vi "Modbus Master.vi"(0 "starting address":u16 caption="起始地址", 1 "error in":errorcluster, 5 "holding register values":u16[](array[numeric]) caption="写入保持寄存器的值", 9 "读取写入选择":string(combo), 11 "Unit ID":u8=1) -> (3 "error out":errorcluster, 4 "仪器状态":u16[](array[numeric]), 6 "试剂余量":u16[](array[numeric]), 8 "输出":T1, 10 "各参数测量间隔":u16[](array[numeric]), 14 "校准点信息":u16[](array[numeric]), 15 "关键参数":u16[](array[numeric]))   [LabVIEW 2016, in "数据传输系统.lvlib"]
uses:
  <vilib>/NI/Modbus Library/API/Modbus API.lvclass/Modbus API.ctl
  <vilib>/NI/Modbus Library/Transmission Data Unit/Transmission Data Unit.lvclass/Transmission Data Unit.ctl
  <vilib>/NI/Modbus Library/API/Master/Set Unit ID.vi
  <vilib>/NI/Modbus Library/Transmission Data Unit/Write Unit ID.vi
  <vilib>/NI/Modbus Library/API/Read Transmission Data Unit.vi
  <vilib>/NI/Modbus Library/API/Write Transmission Data Unit.vi
  <vilib>/NI/Modbus Library/API/master/Modbus Master.lvclass
  E:/Program Files (x86)/National Instruments/LabVIEW 2016/vi.lib/NI/Modbus Library/API/Modbus API.lvclass
  <vilib>/NI/Modbus Library/API/Wrapper/Create TCP Master.vi
  <vilib>/NI/Modbus Library/API/Modbus API.lvclass
  <vilib>/NI/Modbus Library/API/Wrapper/API Main.lvlib
panel:
  out "系统信息":u16[](array[numeric]) caption="校准点信息"
  out "告警信息":u16[](array[numeric]) caption="校准点信息"
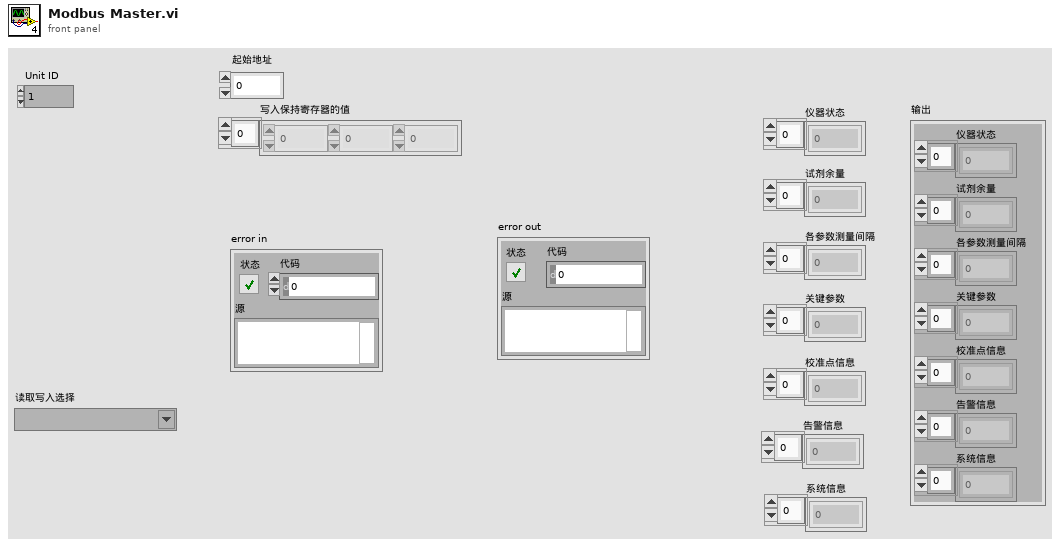
[diagram p1: front panel]
types:
  T1 = cluster{"仪器状态":u16[], "试剂余量":u16[], "各参数测量间隔":u16[], "关键参数":u16[], "校准点信息":u16[], "告警信息":u16[], "系统信息":u16[]}
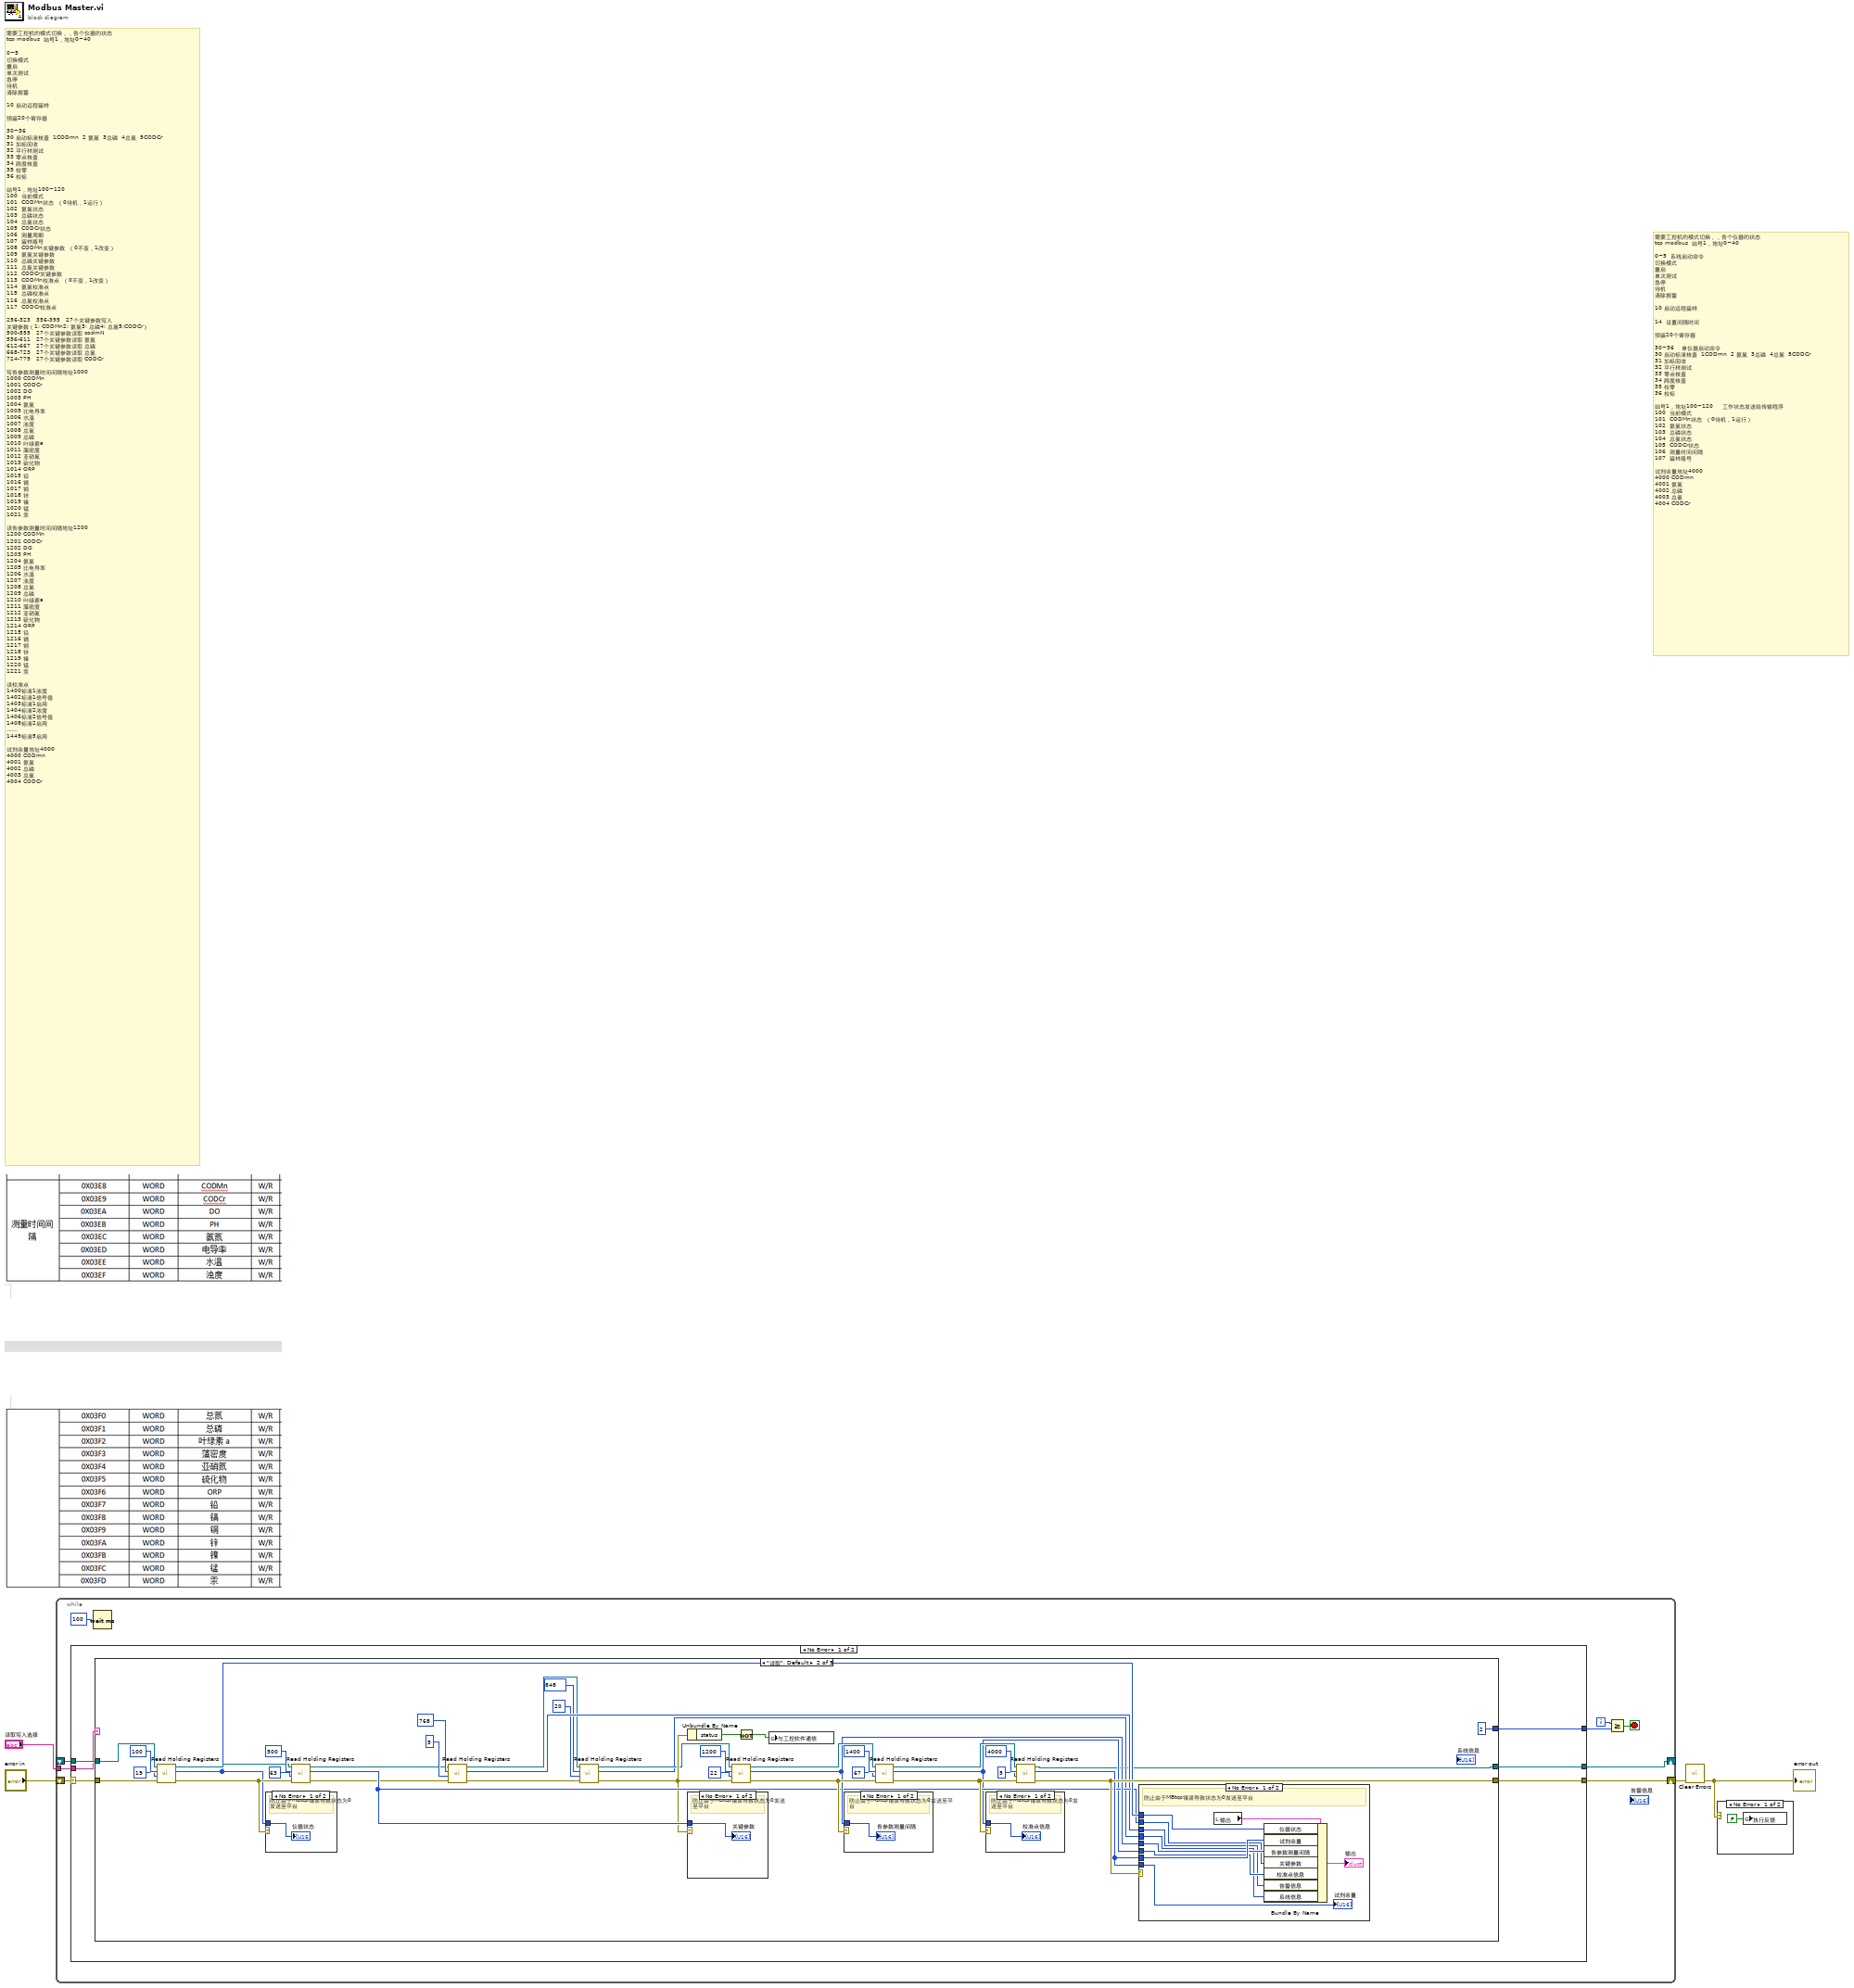
[diagram p0: block diagram]
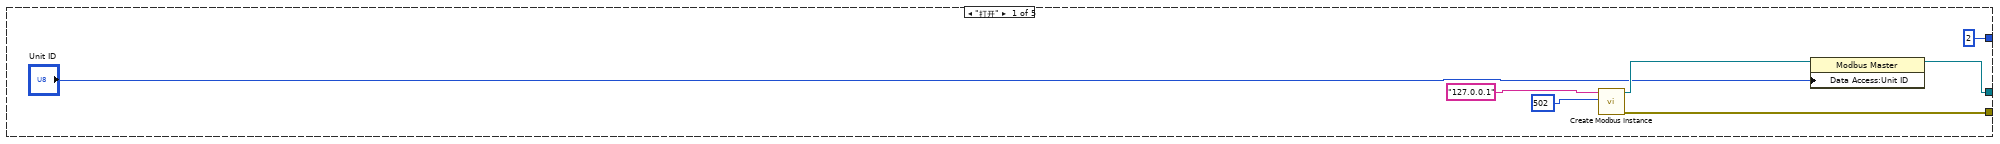
[diagram p3: hidden frame]
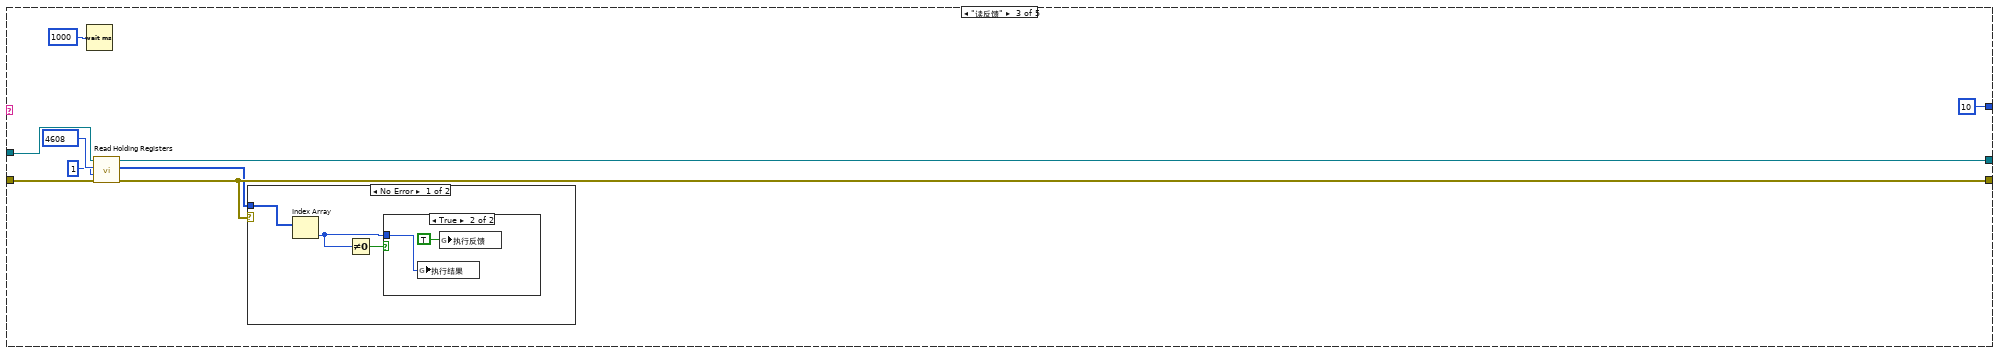
[diagram p9: hidden frame]
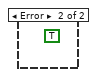
[diagram p11: hidden frame]
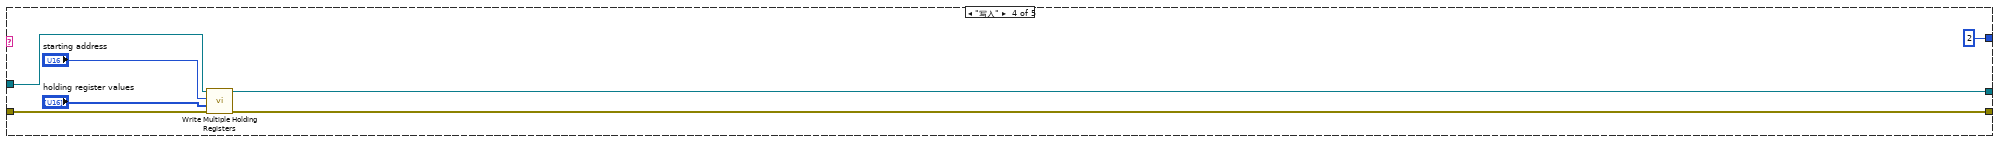
[diagram p12: hidden frame]
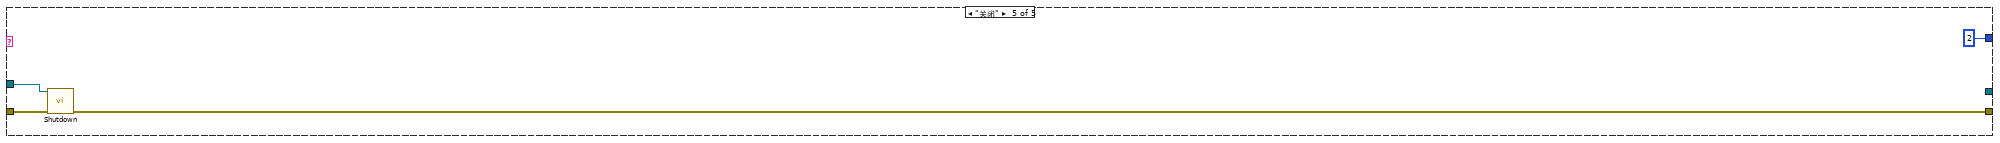
[diagram p13: hidden frame]
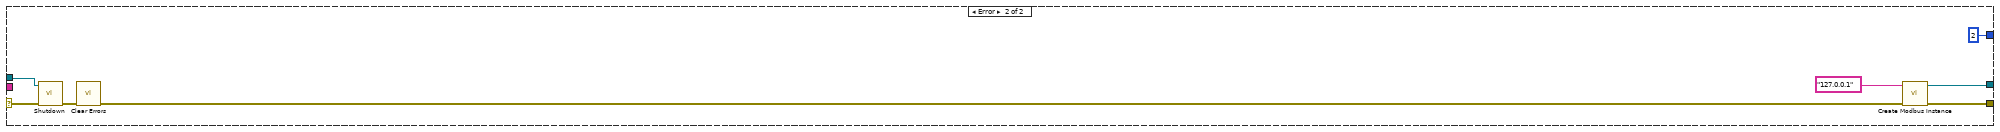
[diagram p14: hidden frame]
diagram:
  # "需要工控机的模式切换，，各个仪器的状态\ntcp modbus  站号1，地址0~40\n\n0~5  系统启动命令\n切换模式\n重启\n单次测试\n急停\n待机\n清除报警\n\n10 启动远程留样\n\n14  设置间隔时间\n\n预留20个寄存器\n\n30~36    单仪器启动命令\n30 启动标液核查  1CODmn  2 氨氮  3总磷  4总氮  5CODCr\n31 加标回收\n32 平行样测试\n33 零点核查\n34 跨度核查\n35 校零\n36 校标\n\n站号1，地址100~120     工作状态发送给传输程序\n100  当前模式\n101  CODMn状态  （0待机，1运行）\n102  氨氮状态\n103  总磷状态\n104  总氮状态\n105  CODCr状态\n106  测量时间间隔\n107  留样瓶号\n\n试剂余量地址4000\n4000 CODmn\n4001 氨氮\n4002 总磷\n4003 总氮\n4004 CODCr"
  # "需要工控机的模式切换，，各个仪器的状态\ntcp modbus  站号1，地址0~40\n\n0~5\n切换模式\n重启\n单次测试\n急停\n待机\n清除报警\n\n10 启动远程留样\n\n预留20个寄存器\n\n30~36\n30 启动标液核查  1CODmn  2 氨氮  3总磷  4总氮  5CODCr\n31 加标回收\n32 平行样测试\n33 零点核查\n34 跨度核查\n35 校零\n36 校标\n\n站号1，地址100~120\n100  当前模式\n101  CODMn状态  （0待机，1运行）\n102  氨氮状态\n103  总磷状态\n104  总氮状态\n105  CODCr状态\n106  测量周期\n107  留样瓶号\n108  CODMn关键参数  （0不变，1改变）\n109  氨氮关键参数\n110  总磷关键参数\n111  总氮关键参数\n112  CODCr关键参数\n113  CODMn校准点  （0不变，1改变）\n114  氨氮校准点\n115  总磷校准点\n116  总氮校准点\n117  CODCr校准点\n\n256-323   356-395   27个关键参数写入\n关键参数（1: CODMn2: 氨氮3: 总磷4: 总氮5:CODCr） \n500-555   27个关键参数读取 codmN\n556-611   27个关键参数读取 氨氮\n612-667   27个关键参数读取 总磷\n668-723   27个关键参数读取 总氮\n724-779   27个关键参数读取 CODCr\n\n写各参数测量时间间隔地址1000\n1000 CODMn\n1001 CODCr\n1002 DO\n1003 PH\n1004 氨氮\n1005 比电导率\n1006 水温\n1007 浊度\n1008 总氮\n1009 总磷\n1010 叶绿素a\n1011 藻密度\n1012 亚硝氮\n1013 硫化物\n1014 ORP\n1015 铅\n1016 镉\n1017 铜\n1018 锌\n1019 镍\n1020 锰\n1021 汞\n\n读各参数测量时间间隔地址1200\n1200 CODMn\n1201 CODCr\n1202 DO\n1203 PH\n1204 氨氮\n1205 比电导率\n1206 水温\n1207 浊度\n1208 总氮\n1209 总磷\n1210 叶绿素a\n1211 藻密度\n1212 亚硝氮\n1213 硫化物\n1214 ORP\n1215 铅\n1216 镉\n1217 铜\n1218 锌\n1219 镍\n1220 锰\n1221 汞\n\n读校准点\n1400标液1浓度\n1402标液1信号值\n1403标液1启用\n1404标液2浓度\n1406标液2信号值\n1408标液2启用\n......\n1449标液5启用\n\n试剂余量地址4000\n4000 CODmn\n4001 氨氮\n4002 总磷\n4003 总氮\n4004 CODCr"
  n1 = while {
    shift-right: [w7] -> w2
    shift-left: "error in" -> [w11]
    shift-right: [w12] -> _
    shift-left: _ -> [w13]
    tunnel: "读取写入选择" -> [w8]
    i -> [w9]
    stop <- w6 stop-if-true
    n2 = case shown="No Error" w11 {
      selector: w11 -> [w16 w107]
      tunnel: w13 -> [w19 w109]
      tunnel: [w18 w111] -> w12
      tunnel: [w17 w110] -> w7
      tunnel: w8 -> [w15 _]
      tunnel: [w14 2 ("y")] -> w5
      frame No Error {
        n3 = case shown="\"读取\", Default" w15 {
          tunnel: w19 -> [_ w66 w87 w101 w105]
          tunnel: [w23 w27 w85 w100 _] -> w18
          tunnel: [w22 w57 w84 w99 w103] -> w17
          tunnel: w16 -> [_ w65 w86 w98 w104]
          tunnel: [2 ("y") 2 ("y") 10 ("y") 2 ("y") 2 ("y")] -> w14
          frame "打开" {
            n4 = call-poly <vilib>:"Create Modbus Instance.vi"("port (502)"=u16 502, "address"="127.0.0.1") -> ("error out"=w22:errorcluster, "TCP master instance"=w26:refnum<class "Modbus Master.lvclass">)  [unwired: 8 in]
            n5 = property class="Modbus Master"(reference=w26, "Data Access:Unit ID"="Unit ID") -> (reference out=w23:refnum<class "Modbus Master.lvclass">)  [unwired: 1 in, 1 out]
          }
          frame "读取", Default {
            n6 = call-dynamic "Read Holding Registers.vi"("error in"=w65, "number of inputs"=u16 19 ("number of holding registers"), "starting address"=u16 100, "Modbus instance in"=w66) -> ("error out"=w51:errorcluster, "register values"=w44:u16[], "Modbus instance out"=w52:refnum<class "Modbus API.lvclass">)  [unwired: 5 in]
            n7 = case shown="No Error" w51 {
              tunnel: w44 -> [w80 _]
              frame No Error {
                # "防止由于MBtcp错误导致状态为0发送至平台"
                "仪器状态" <- w80
              }
              frame Error {
              }
            }
            n8 = call-dynamic "Read Holding Registers.vi"("error in"=w51, "number of inputs"=u16 63 ("number of holding registers"), "starting address"=u16 500, "Modbus instance in"=w52) -> ("error out"=w37:errorcluster, "register values"=w41:u16[], "Modbus instance out"=w36:refnum<class "Modbus API.lvclass">)  [unwired: 5 in]
            n9 = call-dynamic "Read Holding Registers.vi"("error in"=w37, "number of inputs"=u16 5 ("number of holding registers"), "starting address"=u16 768, "Modbus instance in"=w36) -> ("error out"=w31:errorcluster, "register values"=w35:u16[], "Modbus instance out"=w32:refnum<class "Modbus API.lvclass">)  [unwired: 5 in]
            n10 = call-dynamic "Read Holding Registers.vi"("error in"=w31, "number of inputs"=u16 20 ("number of holding registers"), "starting address"=u16 848, "Modbus instance in"=w32) -> ("error out"=w30:errorcluster, "register values"=w28:u16[], "Modbus instance out"=w29:refnum<class "Modbus API.lvclass">)  [unwired: 5 in]
            n11 = Unbundle By Name(w30) -> ("status"=w61:bool)
            n12 = case shown="No Error" w30 {
              tunnel: w41 -> [w68 _]
              frame No Error {
                # "防止由于MBtcp错误导致状态为0发送至平台"
                "关键参数" <- w68
              }
              frame Error {
              }
            }
            n13 = call-dynamic "Read Holding Registers.vi"("error in"=w30, "number of inputs"=u16 22 ("number of holding registers"), "starting address"=u16 1200, "Modbus instance in"=w29) -> ("error out"=w47:errorcluster, "register values"=w42:u16[], "Modbus instance out"=w48:refnum<class "Modbus API.lvclass">)  [unwired: 5 in]
            n14 = Not(x=w61) -> (.not. x?=w60:bool)
            n15 = global write "全局1.vi" "与工控软件通信"(w60) -> ()
            n16 = case shown="No Error" w47 {
              tunnel: w42 -> [w69 _]
              frame No Error {
                # "防止由于MBtcp错误导致状态为0发送至平台"
                "各参数测量间隔" <- w69
              }
              frame Error {
              }
            }
            n17 = call-dynamic "Read Holding Registers.vi"("error in"=w47, "number of inputs"=u16 67 ("number of holding registers"), "starting address"=u16 1400, "Modbus instance in"=w48) -> ("error out"=w45:errorcluster, "register values"=w40:u16[], "Modbus instance out"=w46:refnum<class "Modbus API.lvclass">)  [unwired: 5 in]
            n18 = case shown="No Error" w45 {
              tunnel: w40 -> [w67 _]
              frame No Error {
                # "防止由于MBtcp错误导致状态为0发送至平台"
                "校准点信息" <- w67
              }
              frame Error {
              }
            }
            n19 = call-dynamic "Read Holding Registers.vi"("error in"=w45, "number of inputs"=u16 5 ("number of holding registers"), "starting address"=u16 4000, "Modbus instance in"=w46) -> ("error out"=w57:errorcluster, "register values"=w43:u16[], "Modbus instance out"=w27:refnum<class "Modbus API.lvclass">)  [unwired: 5 in]
            n20 = case shown="No Error" w57 {
              tunnel: w43 -> [w79 _]
              tunnel: w44 -> [w76 _]
              tunnel: w43 -> [w75 _]
              tunnel: w42 -> [w74 _]
              tunnel: w41 -> [w73 _]
              tunnel: w40 -> [w72 _]
              tunnel: w35 -> [w71 _]
              tunnel: w28 -> [w70 _]
              frame No Error {
                # "防止由于MBtcp错误导致状态为0发送至平台"
                n21 = local read "输出"() -> (w77:T1)
                n22 = Bundle By Name(cluster=w77, "仪器状态"=w76, "试剂余量"=w75, "各参数测量间隔"=w74, "关键参数"=w73, "校准点信息"=w72, "告警信息"=w71, "系统信息"=w70) -> (→"输出":T1)
                "试剂余量" <- w79
              }
              frame Error {
              }
            }
          }
          frame "读反馈" {
            n23 = Wait (ms)(milliseconds to wait=u32 1000 ("等待时间（毫秒）")) -> ()  [unwired: 1 out]
            n24 = call-dynamic "Read Holding Registers.vi"("error in"=w86, "number of inputs"=u16 1 ("number of holding registers"), "starting address"=u16 4608, "Modbus instance in"=w87) -> ("error out"=w84:errorcluster, "register values"=w83:u16[], "Modbus instance out"=w85:refnum<class "Modbus API.lvclass">)  [unwired: 5 in]
            n25 = case shown="No Error" w84 {
              tunnel: w83 -> [w92 _]
              frame No Error {
                n26 = Index Array(array=w92) -> (element=w91:u16)  [unwired: 1 in]
                n27 = Not Equal To 0?(x=w91) -> (x != 0?=w90:bool)
                n28 = case shown="True" w90 {
                  tunnel: w91 -> [_ w93]
                  frame False {
                  }
                  frame True {
                    n29 = global write "全局 反控命令枚举.vi" "执行结果"(w93) -> ()
                    n30 = global write "全局 反控命令枚举.vi" "执行反馈"(TRUE ("执行反馈")) -> ()
                  }
                }
              }
              frame Error {
                (unwired) TRUE
              }
            }
          }
          frame "写入" {
            n31 = call-dynamic "Write Multiple Holding Registers.vi"("error in"=w98, "registers to write"="holding register values", "starting address"="starting address", "Modbus instance in"=w101) -> ("error out"=w99:errorcluster, "Modbus instance out"=w100:refnum<class "Modbus API.lvclass">)  [unwired: 6 in]
          }
          frame "关闭" {
            n32 = call-dynamic "Shutdown.vi"("error in"=w104, "Modbus instance in"=w105) -> ("error out"=w103:errorcluster)  [unwired: 9 in]
          }
        }
      }
      frame Error {
        n33 = call-dynamic "Shutdown.vi"("error in"=w107, "Modbus instance in"=w109) -> ("error out"=w108:errorcluster)  [unwired: 9 in]
        n34 = call <vilib>:"Clear Errors.vi"("error in (no error)"=w108) -> ("error out"=w112:errorcluster)  [unwired: 5 in, 1 out]
        n35 = call-poly <vilib>:"Create Modbus Instance.vi"("error in"=w112, "address"="127.0.0.1") -> ("error out"=w110:errorcluster, "TCP master instance"=w111:refnum<class "Modbus Master.lvclass">)  [unwired: 8 in]
      }
    }
    n36 = Wait (ms)(milliseconds to wait=u32 100 ("等待时间（毫秒）")) -> ()  [unwired: 1 out]
    n37 = Greater Or Equal?(x=w9, y=w5) -> (x >= y?=w6:bool)
  }
  n38 = call <vilib>:"Clear Errors.vi"("error in (no error)"=w2) -> ("error out"=w1:errorcluster)  [unwired: 5 in, 1 out]
  "error out" <- w1
  n39 = case shown="No Error" w1 {
    frame No Error {
      n40 = global write "全局 反控命令枚举.vi" "执行反馈"(FALSE ("执行反馈")) -> ()
    }
    frame Error {
    }
  }
